vi "SubscribeSAL.vi"(8 "error in (no error)":errorcluster, 11 "SAL in":refnum<class "SAL.lvclass">) -> (0 "error out":errorcluster, 3 "SAL out":refnum<class "SAL.lvclass">)   [LabVIEW 2016, in "SAL.lvclass"]
uses:
  SAL.lvclass
  SALLV_m1m3/SALLV_m1m3.lvlib
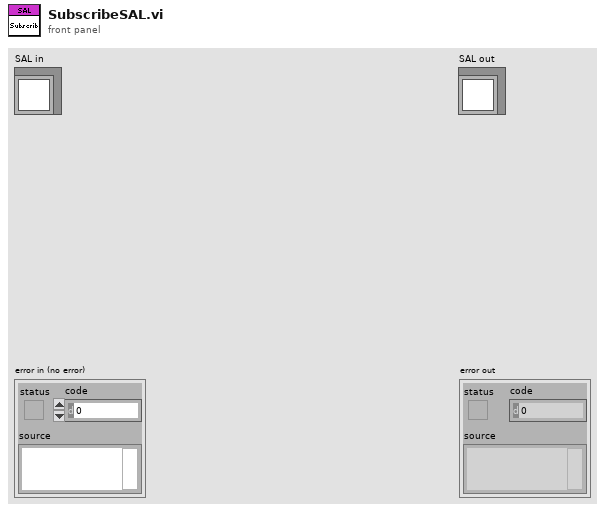
[diagram p1: front panel]
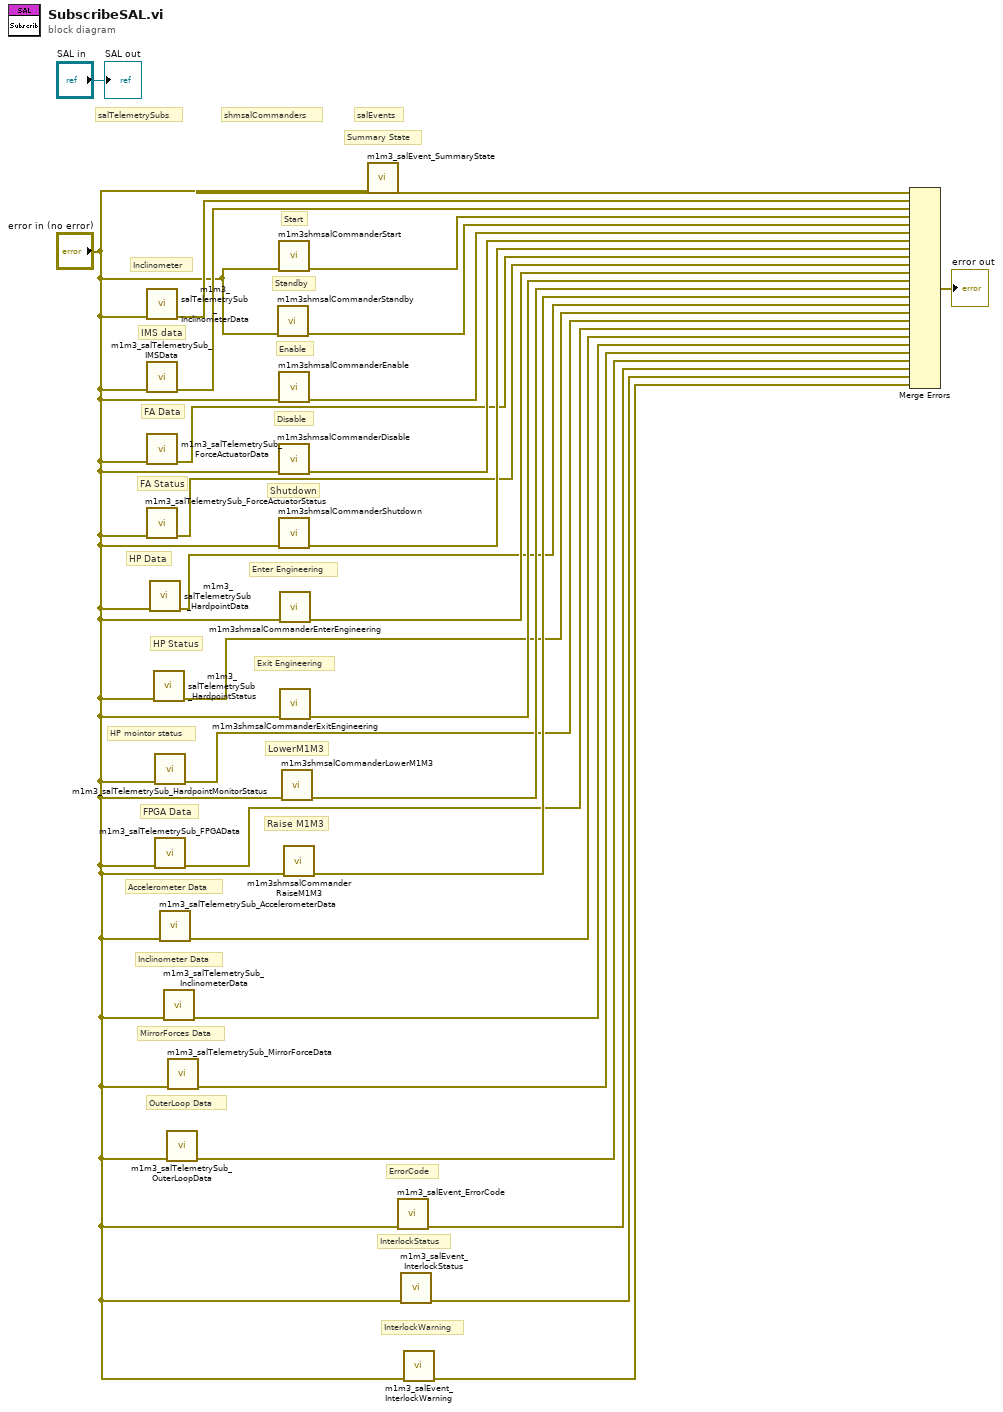
[diagram p0: block diagram]
diagram:
  # "InterlockWarning"
  # "InterlockStatus"
  # "ErrorCode"
  # "salEvents"
  # "OuterLoop Data"
  # "MirrorForces Data"
  # "Inclinometer Data"
  # "Accelerometer Data"
  # "FPGA Data"
  # "HP mointor status"
  # "HP Status"
  # "HP Data"
  # "Raise M1M3"
  # "LowerM1M3"
  # "Exit Engineering"
  # "Enter Engineering"
  # "shmsalCommanders"
  # "salTelemetrySubs"
  # "FA Status"
  # "FA Data"
  # "Shutdown"
  # "Disable"
  # "Enable"
  # "Standby"
  # "Start"
  # "IMS data"
  # "Inclinometer"
  # "Summary State"
  n1 = call "m1m3_salTelemetrySub_InclinometerData.vi"("error in (no error)"="error in (no error)") -> ("error out"=w25:errorcluster)  [unwired: 9 in, 1 out]
  n2 = call "m1m3_salTelemetrySub_IMSData.vi"("error in (no error)"="error in (no error)") -> ("error out"=w24:errorcluster)  [unwired: 9 in, 1 out]
  n3 = call "m1m3_salTelemetrySub_ForceActuatorData.vi"("error in (no error)"="error in (no error)") -> ("error out"=w18:errorcluster)  [unwired: 9 in, 1 out]
  n4 = call "m1m3_salTelemetrySub_ForceActuatorStatus.vi"("error in (no error)"="error in (no error)") -> ("error out"=w17:errorcluster)  [unwired: 9 in, 1 out]
  n5 = call "m1m3_salTelemetrySub_HardpointData.vi"("error in (no error)"="error in (no error)") -> ("error out"=w12:errorcluster)  [unwired: 9 in, 1 out]
  n6 = call "m1m3_salTelemetrySub_HardpointStatus.vi"("error in (no error)"="error in (no error)") -> ("error out"=w11:errorcluster)  [unwired: 9 in, 1 out]
  n7 = call "m1m3_salTelemetrySub_HardpointMonitorStatus.vi"("error in (no error)"="error in (no error)") -> ("error out"=w10:errorcluster)  [unwired: 9 in, 1 out]
  n8 = call "m1m3_salTelemetrySub_FPGAData.vi"("error in (no error)"="error in (no error)") -> ("error out"=w7:errorcluster)  [unwired: 9 in, 1 out]
  n9 = call "m1m3_salTelemetrySub_AccelerometerData.vi"("error in (no error)"="error in (no error)") -> ("error out"=w9:errorcluster)  [unwired: 9 in, 1 out]
  n10 = call "m1m3_salTelemetrySub_InclinometerData.vi"("error in (no error)"="error in (no error)") -> ("error out"=w8:errorcluster)  [unwired: 9 in, 1 out]
  n11 = call "m1m3_salTelemetrySub_OuterLoopData.vi"("error in (no error)"="error in (no error)") -> ("error out"=w5:errorcluster)  [unwired: 9 in, 1 out]
  n12 = call "m1m3_salTelemetrySub_MirrorForceData.vi"("error in (no error)"="error in (no error)") -> ("error out"=w6:errorcluster)  [unwired: 9 in, 1 out]
  n13 = call "m1m3shmsalCommanderStandby.vi"("error in (no error)"="error in (no error)") -> ("error out"=w22:errorcluster)  [unwired: 9 in, 1 out]
  n14 = call "m1m3shmsalCommanderStart.vi"("error in (no error)"="error in (no error)") -> ("error out"=w23:errorcluster)  [unwired: 9 in, 1 out]
  n15 = call "m1m3shmsalCommanderEnable.vi"("error in (no error)"="error in (no error)") -> ("error out"=w21:errorcluster)  [unwired: 9 in, 1 out]
  n16 = call "m1m3shmsalCommanderDisable.vi"("error in (no error)"="error in (no error)") -> ("error out"=w20:errorcluster)  [unwired: 9 in, 1 out]
  n17 = call "m1m3shmsalCommanderShutdown.vi"("error in (no error)"="error in (no error)") -> ("error out"=w19:errorcluster)  [unwired: 9 in, 1 out]
  n18 = call "m1m3shmsalCommanderEnterEngineering.vi"("error in (no error)"="error in (no error)") -> ("error out"=w16:errorcluster)  [unwired: 9 in, 1 out]
  n19 = call "m1m3shmsalCommanderExitEngineering.vi"("error in (no error)"="error in (no error)") -> ("error out"=w15:errorcluster)  [unwired: 9 in, 1 out]
  n20 = call "m1m3shmsalCommanderLowerM1M3.vi"("error in (no error)"="error in (no error)") -> ("error out"=w14:errorcluster)  [unwired: 9 in, 1 out]
  n21 = call "m1m3shmsalCommanderRaiseM1M3.vi"("error in (no error)"="error in (no error)") -> ("error out"=w13:errorcluster)  [unwired: 9 in, 1 out]
  n22 = call "m1m3_salEvent_SummaryState.vi"("error in (no error)"="error in (no error)") -> ("error out"=w27:errorcluster)  [unwired: 9 in, 1 out]
  n23 = call "m1m3_salEvent_ErrorCode.vi"("error in (no error)"="error in (no error)") -> ("error out"=w3:errorcluster)  [unwired: 9 in, 1 out]
  n24 = call "m1m3_salEvent_InterlockStatus.vi"("error in (no error)"="error in (no error)") -> ("error out"=w2:errorcluster)  [unwired: 9 in, 1 out]
  n25 = call "m1m3_salEvent_InterlockWarning.vi"("error in (no error)"="error in (no error)") -> ("error out"=w1:errorcluster)  [unwired: 9 in, 1 out]
  n26 = Merge Errors(w27, w25, w24, w23, w22, w21, w20, w19, w18, w17, w16, w15, w14, w13, w12, w11, w10, w7, w9, w8, w6, w5, w3, w2, w1) -> (→"error out":errorcluster)
  "SAL out" <- "SAL in"
